vi "OnePulseNI.vi"(10 "pulse width ms":u32=1) -> ()   [LabVIEW 2022 SP3]
panel:
  # "configured to use NI  USB-6001 as Dev1\non Analog output channel  0"
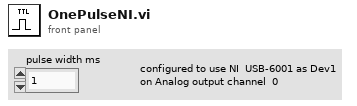
[diagram p1: front panel]
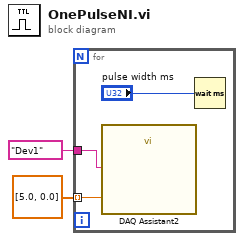
[diagram p0: block diagram]
diagram:
  n1 = for {
    tunnel: dbl[] [5.0, 0.0] -> [w4] mode=indexing
    tunnel: tag "Dev1" ("device name") -> [w3]
    n2 = call "DAQ Assistant2"("data"=w4, "device name"=w3) -> ()  [unwired: 16 in, 2 out]
    n3 = Wait (ms)(milliseconds to wait="pulse width ms") -> ()  [unwired: 1 out]
  }
